vi "Get hours min time.vi"(8 "error in (no error)":errorcluster) -> (0 "error out":errorcluster, 1 "Seconds":string, 2 "Minutes":string, 3 "Hours":string, 4 "AM or PM":string, 5 "24 hr clock hours":string, 6 "24hr time":string)   [LabVIEW 2013]
panel:
  out "time string":string
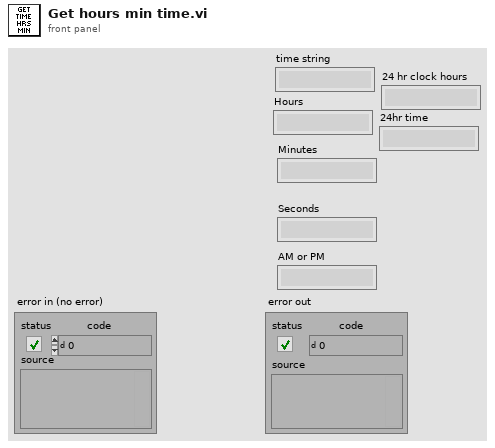
[diagram p1: front panel]
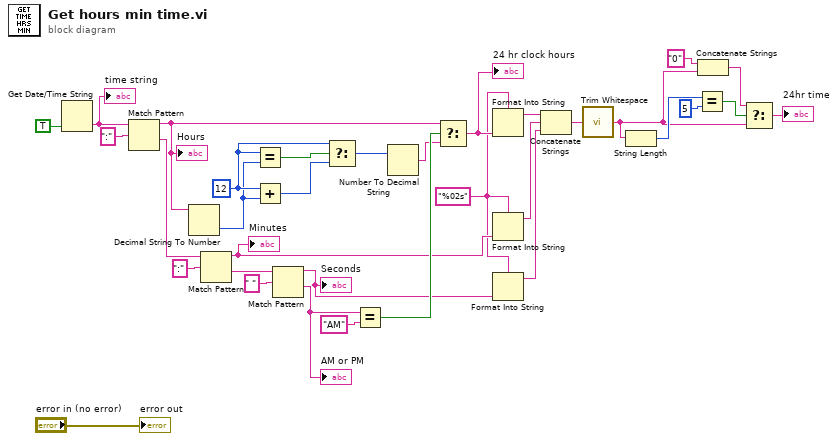
[diagram p0: block diagram]
diagram:
  w10 = "%02s" ("format string")
  w19 = 12 ("x")
  n1 = Get Date/Time String(want seconds? (F)=TRUE) -> (time string=w33:string)  [unwired: 2 in, 1 out]
  "time string" <- w33
  n2 = Match Pattern(string=w33, regular expression=":") -> (before substring=w21:string, after substring=w28:string)  [unwired: 1 in, 2 out]
  "Hours" <- w21
  n3 = Decimal String To Number(string=w21) -> (number=w18:i32)  [unwired: 2 in, 1 out]
  n4 = Match Pattern(string=w28, regular expression=":") -> (before substring=w13:string, after substring=w27:string)  [unwired: 1 in, 2 out]
  "Minutes" <- w13
  n5 = Equal?(x=w19, y=w18) -> (x = y?=w22:bool)
  n6 = Add(x=w19, y=w18) -> (x+y=w20:i32)
  n7 = Match Pattern(string=w27, regular expression=" ") -> (before substring=w11:string, after substring=w25:string)  [unwired: 1 in, 2 out]
  "AM or PM" <- w25
  "Seconds" <- w11
  n8 = Select(t=w19, s=w22, f=w20) -> (s? t:f=w17:i32)
  n9 = Equal?(x=w25, y="AM") -> (x = y?=w23:bool)
  n10 = Number To Decimal String(number=w17) -> (decimal integer string=w16:string)  [unwired: 1 in]
  n11 = Select(t=w21, s=w23, f=w16) -> (s? t:f=w15:string)
  "24 hr clock hours" <- w15
  n12 = Format Into String(format string=w10, w15) -> (resulting string=w14:string)  [unwired: 2 in, 1 out]
  n13 = Format Into String(format string=w10, w13) -> (resulting string=w12:string)  [unwired: 2 in, 1 out]
  n14 = Format Into String(format string=w10, w11) -> (resulting string=w9:string)  [unwired: 2 in, 1 out]
  n15 = Concatenate Strings(w14, w12, w9) -> (w2:string)
  n16 = call <vilib>:"Trim Whitespace.vi"("string"=w2) -> ("trimmed string"=w1:string)  [unwired: 1 in]
  n17 = String Length(string=w1) -> (length=w8:i32)
  n18 = Equal?(x=w8, y=5) -> (x = y?=w6:bool)
  n19 = Concatenate Strings("0" ("string"), w1) -> (w4:string)
  n20 = Select(t=w4, s=w6, f=w1) -> (s? t:f=→"24hr time":string)
  "error out" <- "error in (no error)"
